vi "segment.vi"(8 "error in (no error)":errorcluster, 9 "ImageCollection in":refnum<class "ImageCollection.lvclass">[](array[class]), 10 "image file path":path, 11 "SegmenterMG100305SingleCell in":refnum<class "SegmenterMG100305SingleCell.lvclass">) -> (0 "error out":errorcluster, 1 "ImageCollection out":refnum<class "ImageCollection.lvclass">[](array[class]), 2 "segmented image path out":path, 3 "SegmenterMG100305SingleCell out":refnum<class "SegmenterMG100305SingleCell.lvclass">, 4 "centroids":T3[](array[typedef]))   [LabVIEW 2010, in "SegmenterMG100305SingleCell.lvclass"]
uses:
  SegmenterMG100305SingleCell.lvclass
  common/classes/ImageCollection/ImageCollection/ImageCollection.lvclass
  <vilib>/vision/Image Controls.llb/IMAQ Image.ctl
  GenericSegmenter/GenericSegmenter/centroid_cluster.ctl
  common/classes/ImageCollection/ImageCollection/add_mode_enum.ctl
  common/classes/Image/Image/Image.lvclass
  <vilib>/vision/Image Controls.llb/IMAQ Rounding Mode.ctl
  <vilib>/Utility/inputDevices.llb/mouseAcquire.vi
  <vilib>/vision/NI_Vision_Development_Module.lvlib
  GenericSegmenter/GenericSegmenter/GenericSegmenter.lvclass
panel:
  out "Image 2":T1(plugin-control)
  out "Intensity Graph":u8[][](graph)
  out "XY Graph":cluster{"x":i32, "y":i32}[](graph)
  out "ROI":T2
  out "Image Dst Out":T1
  in  "done button":bool
  in  "Threshold Values":T4(slide)={"Minimum Value"=0.0, "Maximum Value"=135.0} scale=0.0..255.0
  out "Image":T1(plugin-control)
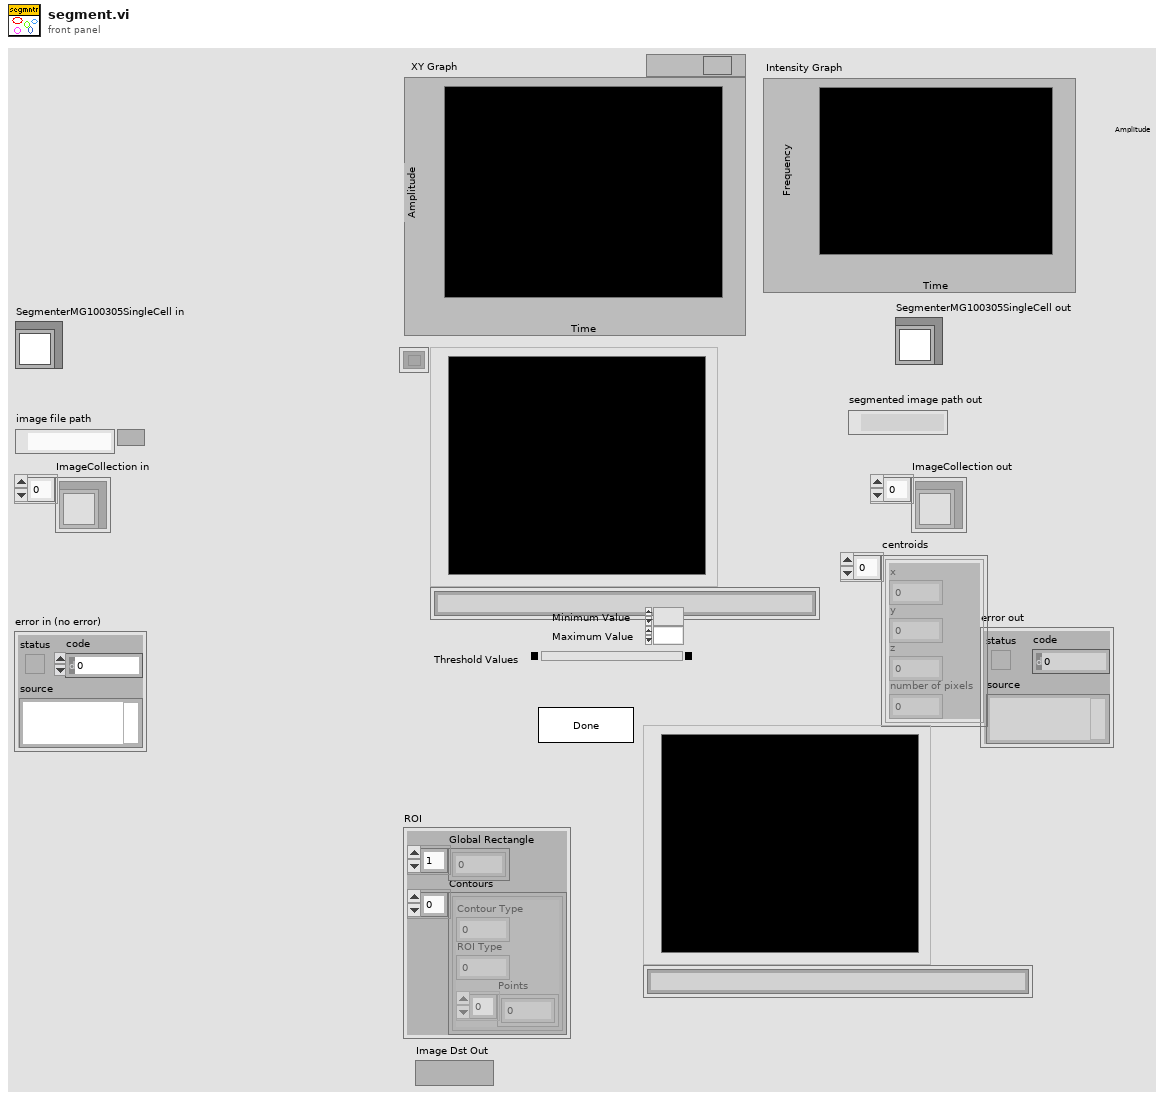
[diagram p1: front panel]
types:
  T1 = typedef "IMAQ Image.ctl" = refnum<image>
  T2 = cluster{"Global Rectangle":i32[], "Contours":cluster{"Contour Type":u32, "ROI Type":u32, "Points":i32[]}[]}
  T3 = typedef "GenericSegmenter.lvclass/centroid_cluster.ctl" = cluster{"x":i32, "y":i32, "z":i32, "number of pixels":i32}
  T4 = cluster{"Minimum Value":sgl, "Maximum Value":sgl}
  T5 = enum8{"Enabled", "Disabled", "Disabled and Grayed Out"}
  T6 = typedef "ImageCollection.lvclass/add_mode_enum.ctl" = enum16{"instance", "copy"}
  T7 = typedef "IMAQ Rounding Mode.ctl" = enum16{"Optimize", "Truncate"}
  T8 = enum32{"AutoM", "Close", "Dilate", "Erode", "Gradient", "Gradient out", "Gradient in", "Hit miss", "Open", "PClose", "POpen", "Thick", "Thin"}
  T9 = typedef "Image Type" = u32
  T10 = cluster{"Horizontal":i32, "Vertical":i32, "Scrolling":i32}
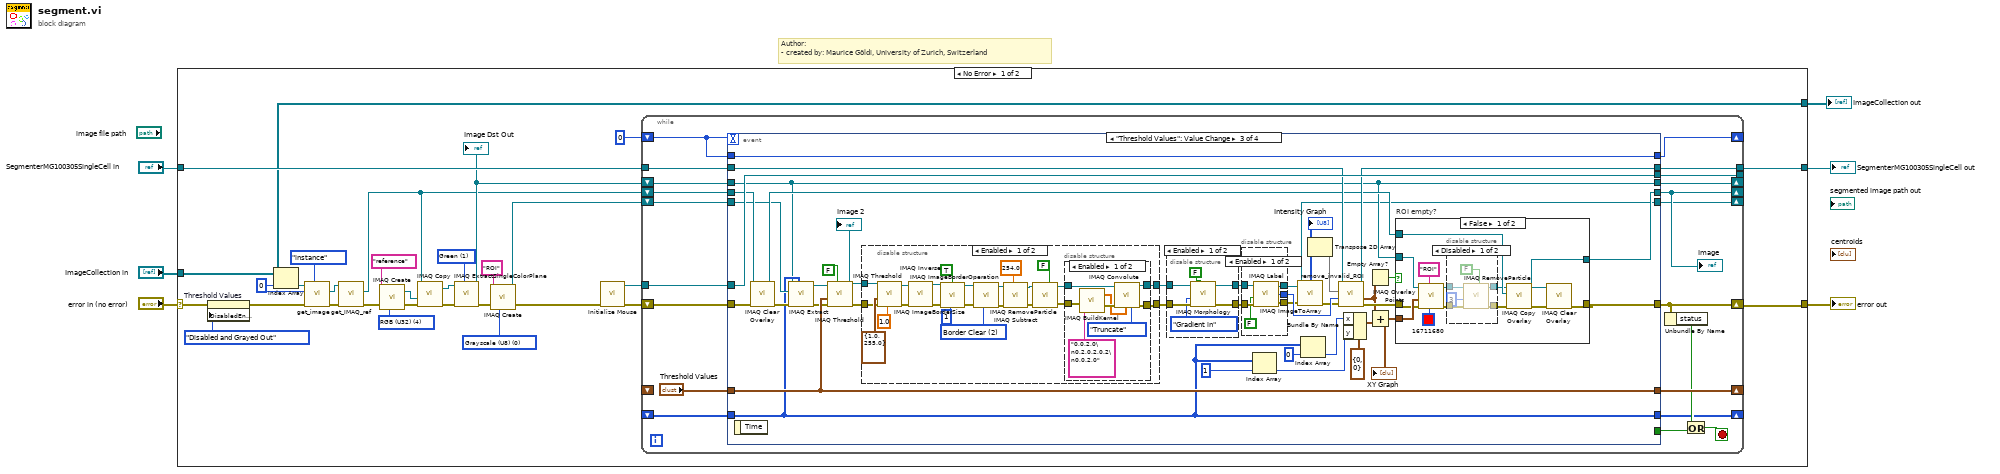
[diagram p0: block diagram]
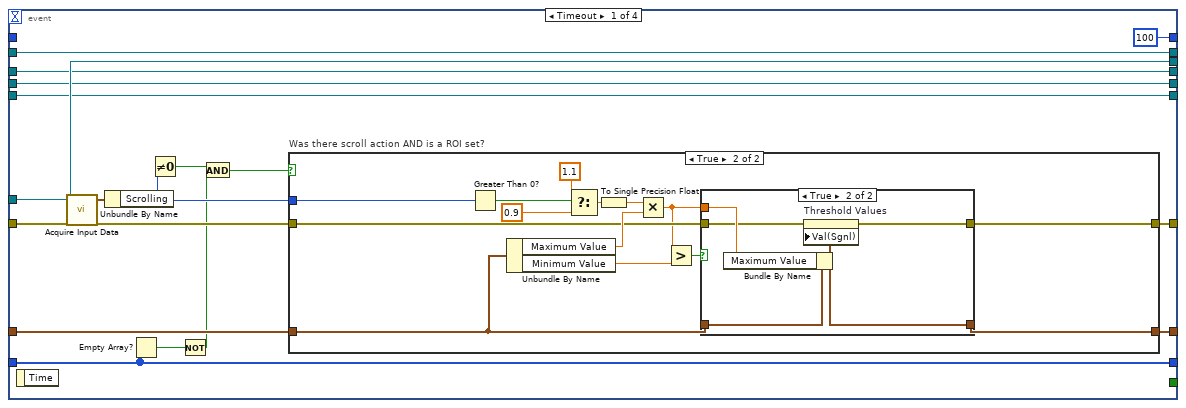
[diagram p2: hidden frame]
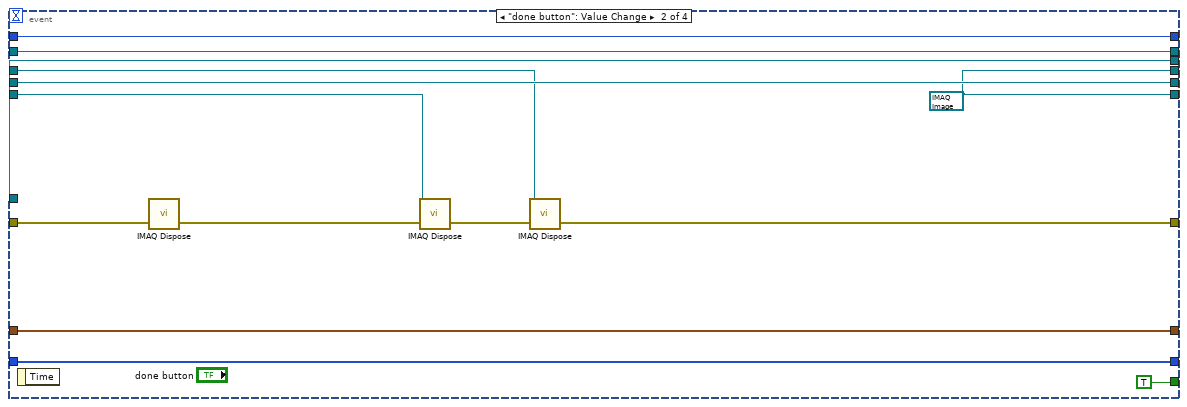
[diagram p5: hidden frame]
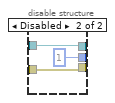
[diagram p6: hidden frame]
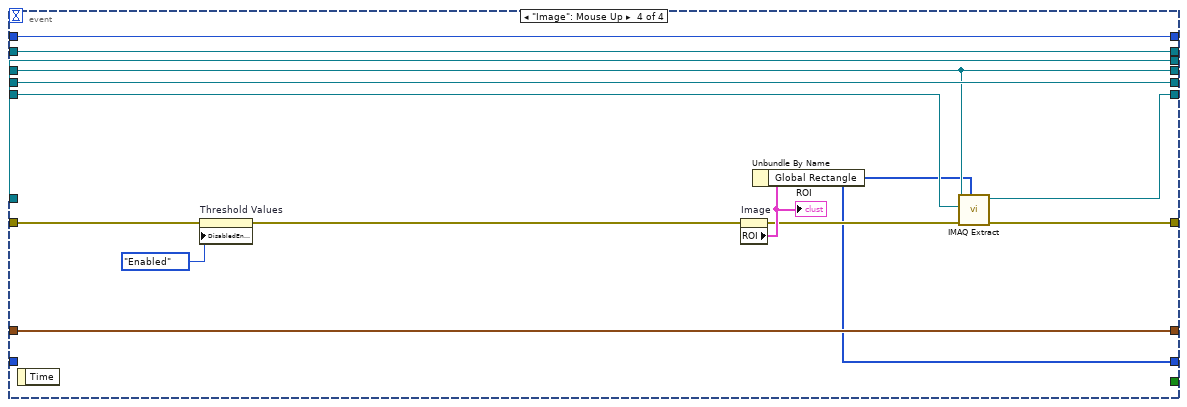
[diagram p12: hidden frame]
diagram:
  # "Author: \n- created by: Maurice Göldi, University of Zurich, Switzerland"
  n1 = case shown="No Error" "error in (no error)" {
    selector: "error in (no error)" -> [w11 w245]
    tunnel: [w27 w245] -> w5
    tunnel: "ImageCollection in" -> [w25 w244]
    tunnel: [w26 w243] -> w3
    tunnel: "SegmenterMG100305SingleCell in" -> [w31 w243]
    tunnel: [w25 w244] -> w1
    frame No Error {
      w8 = T9 0 items=["Grayscale (U8)", "Grayscale (I16)", "Grayscale (SGL)", "Complex (CSG)", "RGB (U32)", "HSL (U32)", "RGB (U64)", "Grayscale (U16)"] ("Image Type")
      w14 = T9 4 items=["Grayscale (U8)", "Grayscale (I16)", "Grayscale (SGL)", "Complex (CSG)", "RGB (U32)", "HSL (U32)", "RGB (U64)", "Grayscale (U16)"] ("Image Type")
      w24 = 1 items=["Red", "Green", "Blue", "Hue", "Saturation", "Luminance", "Value", "Intensity"] ("Color Plane")
      w35 = 0 ("index")
      n2 = property on="Threshold Values" class="Slide (strict)"(error in=w11, "DisabledEnum"=T5."Disabled and Grayed Out" ("Disabled")) -> (error out=w10:errorcluster)  [unwired: 1 in, 1 out]
      n3 = Index Array(array=w25, index=w35) -> (element=w36:refnum<class "ImageCollection.lvclass">)
      n4 = call-dynamic "get_image.vi"("get image as..."=add_mode_enum."instance", "error in (no error)"=w10, "index"=w35, "ImageCollection in"=w36) -> ("error out"=w33:errorcluster, "Image.lvclass"=w32:refnum<class "Image.lvclass">)  [unwired: 5 in, 1 out]
      n5 = call-dynamic "get_IMAQ_ref.vi"("error in (no error)"=w33, "Image.lvclass in"=w32) -> ("error out"=w23:errorcluster, "Image"=w17:T1)  [unwired: 5 in, 3 out]
      n6 = call "IMAQ Create"("Image Name"="reference", "Image Type"=w14, "error in (no error)"=w23) -> ("New Image"=w18:T1, "error out"=w20:errorcluster)  [unwired: 2 in]
      n7 = call "IMAQ Copy"("error in (no error)"=w20, "Image Dst"=w18, "Image Src"=w17) -> ("error out"=w19:errorcluster, "Image Dst Out"=w16:T1)  [unwired: 3 in]
      n8 = call "IMAQ ExtractSingleColorPlane"("Color Plane"=w24, "error in (no error)"=w19, "Image Src"=w16) -> ("error out"=w15:errorcluster, "Image Dst Out"=w22:T1)  [unwired: 7 in]
      "Image Dst Out" <- w22
      n9 = call "IMAQ Create"("Image Name"="ROI", "Image Type"=w8, "error in (no error)"=w15) -> ("New Image"=w12:T1, "error out"=w7:errorcluster)  [unwired: 2 in]
      n10 = call <vilib>:"Initialize Mouse.vi"("error in (no error)"=w7) -> ("error out"=w29:errorcluster, "device ID"=w28:refnum<k1>)  [unwired: 9 in]
      n11 = while {
        tunnel: w31 -> [w50]
        tunnel: w28 -> [w56]
        tunnel: [w55] -> _
        shift-right: [w54] -> _
        shift-left: 0 -> [w57]
        shift-right: [w47] -> w27
        shift-left: w29 -> [w53]
        shift-right: [w51] -> _
        shift-left: _ -> [_]
        tunnel: [w49] -> w26
        shift-right: [w48] -> _
        shift-left: w17 -> [w37]
        shift-right: [w43] -> _
        shift-left: w22 -> [w44]
        shift-right: [w41] -> _
        shift-left: w12 -> [w42]
        shift-right: [w39] -> _
        shift-left: _ -> [w38]
        stop <- w45 stop-if-true
        n12 = event shown="[2] \"Threshold Values\": Value Change" {
          selector: _ -> [_ _ _ _]
          dyn-events: _ -> [_ _ _ _]
          timeout: w57 -> [_ _ _ _]
          tunnel: w57 -> [_ w112 w151 w241]
          tunnel: w56 -> [w74 w113 w152 w242]
          tunnel: [w73 w113 w152 w242] -> w55
          tunnel: [100 w112 w151 w241] -> w54
          tunnel: [w71 w107 w145 w236] -> w47
          tunnel: w53 -> [w75 w102 w142 w233]
          tunnel: "Threshold Values" -> [w70 w109 w147 w240]
          tunnel: [w68 w109 w147 w240] -> w51
          tunnel: w37 -> [w66 w110 w141 w235]
          tunnel: w50 -> [w67 w111 w149 w239]
          tunnel: [w67 w111 w148 w239] -> w49
          tunnel: [w66 w110 w143 w235] -> w48
          tunnel: w44 -> [w65 w105 w123 w230]
          tunnel: [w65 w100 w123 w230] -> w43
          tunnel: w42 -> [w64 w106 w129 w234]
          tunnel: [w64 w100 w120 w228] -> w41
          tunnel: [_ TRUE _ _] -> w40
          tunnel: [w61 w103 w127 w229] -> w39
          tunnel: w38 -> [w61 w103 w127 _]
          event Timeout {
            n13 = event-data() -> ()  [unwired: 1 in, 1 out]
            n14 = call-poly <vilib>:"Acquire Input Data.vi"("device ID"=w74, "error in (no error)"=w75) -> ("device ID"=w73:refnum<k1>, "axis info"=w72:T10, "error out"=w60:errorcluster)  [unwired: 14 in, 1 out]
            n15 = Unbundle By Name(w72) -> ("Scrolling"=w69:i32)
            n16 = Empty Array?(array=w61) -> (empty?=w58:bool)
            n17 = Not Equal To 0?(x=w69) -> (x != 0?=w63:bool)
            n18 = Not(x=w58) -> (.not. x?=w59:bool)
            n19 = And(x=w63, y=w59) -> (x .and. y?=w62:bool)
            n20 = case "Was there scroll action AND is a ROI set?" shown="True" w62 {
              tunnel: w60 -> [w78 w88]
              tunnel: [w78 w87] -> w71
              tunnel: w69 -> [_ w92]
              tunnel: w70 -> [w77 w89]
              tunnel: [w77 w86] -> w68
              frame False {
              }
              frame True {
                n21 = Greater Than 0?(x=w92) -> (x > 0?=w91:bool)
                n22 = Unbundle By Name(w89) -> ("Maximum Value"=w90:sgl, "Minimum Value"=w80:sgl)
                n23 = Select(t=1.1, s=w91, f=0.9) -> (s? t:f=w83:dbl)
                n24 = To Single Precision Float(number=w83) -> (single precision float=w82:sgl)
                n25 = Multiply(x=w82, y=w90) -> (x*y=w79:sgl)
                n26 = Greater?(x=w79, y=w80) -> (0:w81:bool)
                n27 = case shown="True" w81 {
                  tunnel: w89 -> [w93 w99]
                  tunnel: w79 -> [_ w98]
                  tunnel: w88 -> [w94 w97]
                  tunnel: [w94 w96] -> w87
                  tunnel: [w93 w95] -> w86
                  frame False {
                  }
                  frame True {
                    n28 = Bundle By Name(cluster=w99, "Maximum Value"=w98) -> (w95:T4)
                    n29 = property on="Threshold Values" class="Slide (strict)"(error in=w97, "Val(Sgnl)"=w95) -> (error out=w96:errorcluster)  [unwired: 1 in, 1 out]
                  }
                }
              }
            }
          }
          event "done button": Value Change {
            w100 = T1 refnum ("New Image")
            n30 = event-data() -> ()  [unwired: 1 in, 1 out]
            n31 = call "IMAQ Dispose"("error in (no error)"=w102) -> ("error out"=w101:errorcluster)  [unwired: 5 in]
            n32 = call "IMAQ Dispose"("Image"=w106, "error in (no error)"=w101) -> ("error out"=w108:errorcluster)  [unwired: 4 in]
            n33 = call "IMAQ Dispose"("Image"=w105, "error in (no error)"=w108) -> ("error out"=w107:errorcluster)  [unwired: 4 in]
          }
          event "Threshold Values": Value Change {
            n34 = event-data() -> ()  [unwired: 1 in, 1 out]
            n35 = call "IMAQ Clear Overlay"("error in (no error)"=w142, "Image"=w141) -> ("error out"=w131:errorcluster, "Image Out"=w140:T1)  [unwired: 8 in]
            n36 = call "IMAQ Extract"("Optional Rectangle"=w127, "error in (no error)"=w131, "Image Dst"=w129, "Image Src"=w123) -> ("error out"=w130:errorcluster, "Image Dst Out"=w128:T1)  [unwired: 6 in]
            n37 = call "IMAQ Threshold"("Keep/Replace Value (Replace)"=FALSE, "error in (no error)"=w130, "Range"=w147, "Image Src"=w128) -> ("error out"=w118:errorcluster, "Image Dst Out"=w119:T1)  [unwired: 6 in]
            "Image 2" <- w119
            n38 = disable-structure shown="Enabled" {
              disable-tunnel: w119 -> [w180 w196]
              disable-tunnel: w118 -> [w179 w195]
              disable-tunnel: [w171 w195] -> w117
              disable-tunnel: [w170 w196] -> w116
              frame Enabled {
                w174 = u32 2 items=["Border Mirror", "Border Copy", "Border Clear"] ("Function")
                n39 = call "IMAQ Threshold"("Replace Value"=sgl 1.0, "error in (no error)"=w179, "Range"=cluster{"Lower value":sgl, "Upper value":sgl} {"Lower value"=1.0, "Upper value"=255.0}, "Image Src"=w180) -> ("error out"=w184:errorcluster, "Image Dst Out"=w183:T1)  [unwired: 6 in]
                n40 = call "IMAQ Inverse"("error in (no error)"=w184, "Image Src"=w183) -> ("error out"=w173:errorcluster, "Image Dst Out"=w172:T1)  [unwired: 8 in]
                n41 = call "IMAQ ImageBorderSize"("Get/Set Status? (Set)"=TRUE, "Image"=w172, "Image border size in"=1, "error in (no error)"=w173) -> ("Image Out"=w177:T1, "error out"=w178:errorcluster)  [unwired: 1 out]
                n42 = call "IMAQ ImageBorderOperation"("Image"=w177, "Function"=w174, "error in (no error)"=w178) -> ("Image Out"=w168:T1, "error out"=w169:errorcluster)  [unwired: 2 in]
                n43 = call "IMAQ Subtract"("Image Src A"=w168, "Constant"=sgl 254.0, "error in (no error)"=w169) -> ("Image Dst Out"=w166:T1, "error out"=w164:errorcluster)  [unwired: 4 in]
                n44 = call "IMAQ RemoveParticle"("Connectivity 4/8 (8)"=FALSE, "error in (no error)"=w164, "Image Src"=w166) -> ("error out"=w163:errorcluster, "Image Dst Out"=w165:T1)  [unwired: 7 in]
                n45 = disable-structure shown="Enabled" {
                  disable-tunnel: [w188 w193] -> w171
                  disable-tunnel: [w187 w194] -> w170
                  disable-tunnel: w163 -> [w186 w193]
                  disable-tunnel: w165 -> [w185 w194]
                  frame Enabled {
                    n46 = call "IMAQ BuildKernel"("Kernel String"="0,0.2,0\n0.2,0.2,0.2\n0,0.2,0", "error in (no error)"=w186) -> ("Kernel"=w191:sgl[][], "error out"=w192:errorcluster)  [unwired: 3 in]
                    n47 = call "IMAQ Convolute"("Rounding Mode"=IMAQ_Rounding_Mode."Truncate", "Kernel"=w191, "error in (no error)"=w192, "Image Src"=w185) -> ("error out"=w188:errorcluster, "Image Dst Out"=w187:T1)  [unwired: 6 in]
                  }
                  frame Disabled {
                  }
                }
              }
              frame Disabled {
              }
            }
            n48 = disable-structure shown="Enabled" {
              disable-tunnel: [w202 w204] -> w115
              disable-tunnel: [w201 w203] -> w114
              disable-tunnel: w117 -> [w200 w203]
              disable-tunnel: w116 -> [w199 w204]
              frame Enabled {
                n49 = call "IMAQ Morphology"("Square/Hexa (Square)"=FALSE, "error in (no error)"=w200, "Operation"=T8."Gradient in", "Image Src"=w199) -> ("error out"=w201:errorcluster, "Image Dst Out"=w202:T1)  [unwired: 6 in]
              }
              frame Disabled {
              }
            }
            n50 = disable-structure shown="Enabled" {
              disable-tunnel: [w158 1 ("number of particles")] -> w150
              disable-tunnel: [w157 w161] -> w121
              disable-tunnel: [w156 w160] -> w120
              disable-tunnel: w115 -> [w155 w160]
              disable-tunnel: w114 -> [w154 w161]
              frame Enabled {
                n51 = call "IMAQ Label"("error in (no error)"=w154, "Connectivity 4/8 (8)"=FALSE, "Image Src"=w155) -> ("error out"=w157:errorcluster, "Number of Particles"=w158:i32, "Image Dst Out"=w156:T1)  [unwired: 1 in]
              }
              frame Disabled {
              }
            }
            n52 = Index Array(array=w127, index=1) -> (element=w134:i32)
            n53 = call "IMAQ ImageToArray"("error in (no error)"=w121, "Image"=w120) -> ("error out"=w124:errorcluster, "Image Pixels (U8)"=w122:u8[][])  [unwired: 2 in, 3 out]
            "Intensity Graph" <- w122
            n54 = Index Array(array=w127, index=0) -> (element=w135:i32)
            n55 = Transpose 2D Array(2D array=w122) -> (transposed array=w125:u8[][])
            n56 = call-dynamic "remove_invalid_ROI.vi"("error in (no error)"=w124, "number of particles"=w150, "Image Pixels in"=w125, "SegmenterMG100305SingleCell in"=w149) -> ("error out"=w146:errorcluster, "ROI array out"=w132:cluster{"x":i32, "y":i32}[], "SegmenterMG100305SingleCell out"=w148:refnum<class "SegmenterMG100305SingleCell.lvclass">)  [unwired: 4 in, 1 out]
            n57 = Bundle By Name(cluster=cluster{"x":i32, "y":i32} {"x"=0, "y"=0} ("point"), "x"=w135, "y"=w134) -> (w138:cluster{"x":i32, "y":i32})
            n58 = Empty Array?(array=w132) -> (empty?=w144:bool)
            n59 = Add(x=w132, y=w138) -> (x+y=w133:cluster{"x":i32, "y":i32}[])
            "XY Graph" <- w133
            n60 = case "ROI empty?" shown="False" w144 {
              tunnel: w146 -> [w214 w227]
              tunnel: [w207 w227] -> w145
              tunnel: w133 -> [w217 _]
              tunnel: w140 -> [w209 w226]
              tunnel: [w205 w226] -> w143
              tunnel: w123 -> [w211 _]
              frame False {
                n61 = call "IMAQ Overlay Points"("Color"=u32 16711680, "Group"="ROI", "error in (no error)"=w214, "Array of Points"=w217, "Image"=w211) -> ("error out"=w213:errorcluster, "Image Out"=w212:T1)  [unwired: 5 in]
                n62 = disable-structure shown="Disabled" {
                  disable-tunnel: w213 -> [w223 w225]
                  disable-tunnel: w212 -> [w222 w224]
                  disable-tunnel: [w221 w225] -> w210
                  disable-tunnel: [w220 w224] -> w206
                  frame Disabled {
                    n63 = call "IMAQ RemoveParticle"("Connectivity 4/8 (8)"=FALSE ("Square/Hexa (Square)"), "error in (no error)"=w223, "Number of Erosion"=3, "Image Src"=w222) -> ("error out"=w221:errorcluster, "Image Dst Out"=w220:T1)  [unwired: 6 in]
                  }
                  frame Enabled {
                  }
                }
                n64 = call "IMAQ Copy Overlay"("error in (no error)"=w210, "Image Dst"=w209, "Image Src"=w206) -> ("error out"=w208:errorcluster, "Image Dst Out"=w205:T1)  [unwired: 7 in]
                n65 = call "IMAQ Clear Overlay"("error in (no error)"=w208, "Image"=w206) -> ("error out"=w207:errorcluster)  [unwired: 8 in, 1 out]
              }
              frame True {
              }
            }
          }
          event "Image": Mouse Up {
            n66 = event-data() -> ()  [unwired: 1 in, 1 out]
            n67 = property on="Threshold Values" class="Slide (strict)"(error in=w233, "DisabledEnum"=T5."Enabled" ("Disabled")) -> (error out=w232:errorcluster)  [unwired: 1 in, 1 out]
            n68 = property on="Image" class="ImageControl"(error in=w232) -> (error out=w237:errorcluster, "ROI"=w238:T2)  [unwired: 1 in, 1 out]
            "ROI" <- w238
            n69 = Unbundle By Name(w238) -> ("Global Rectangle"=w229:i32[])
            n70 = call "IMAQ Extract"("Optional Rectangle"=w229, "error in (no error)"=w237, "Image Dst"=w234, "Image Src"=w230) -> ("error out"=w236:errorcluster, "Image Dst Out"=w228:T1)  [unwired: 6 in]
          }
        }
        "Image" <- w48
        n71 = Unbundle By Name(w47) -> ("status"=w46:bool)
        n72 = Or(x=w46, y=w40) -> (x .or. y?=w45:bool)
      }
    }
    frame Error {
    }
  }
  "error out" <- w5
  "SegmenterMG100305SingleCell out" <- w3
  "ImageCollection out" <- w1
